vi "onProcessStopped.vi"(8 "error in (no error)":errorcluster, 11 "SystemController":refnum<class "SystemController.lvclass">) -> (0 "error out":errorcluster, 3 "SystemController out":refnum<class "SystemController.lvclass">)   [LabVIEW 2017, in "SystemController.lvclass"]
doc: "JKI State Machine Objects (SMO) 1.3.0.56\nJKI - JKI\nCopyright (c) 2017, JKI"
uses:
  SystemController.lvclass
  Camera/Camera_class/Camera.lvclass
  ImageFacialDetection_class/ImageFacialDetection.lvclass
  <vilib>/JKI/JKI SMO/SMO/SMO.lvclass
panel:
  # "For instructions on how to use the JKI State Machine Objects, examples and video tutorials, visit:\nhttp://jki.net/state-machine-objects/\n\nJKI State Machine Objects™\nhttp://jki.net/state-machine-objects/\nCopyright (C) 2005-2015, JKI <info@jki.net>\nALL RIGHTS RESERVED"
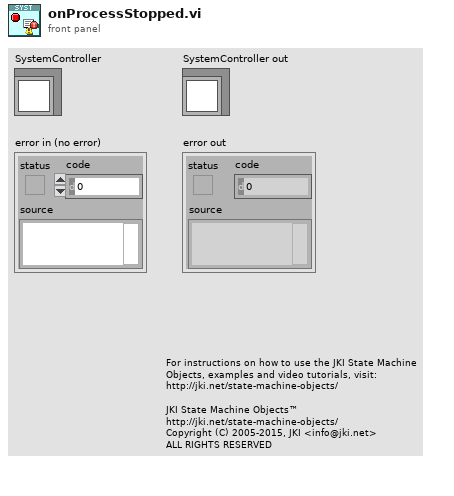
[diagram p1: front panel]
types:
  T1 = typedef "SystemController.lvclass/Dependencies--Cluster.ctl" = cluster{"Camera":refnum<class "Camera.lvclass">, "ImageFacialDetection":refnum<class "ImageFacialDetection.lvclass">}
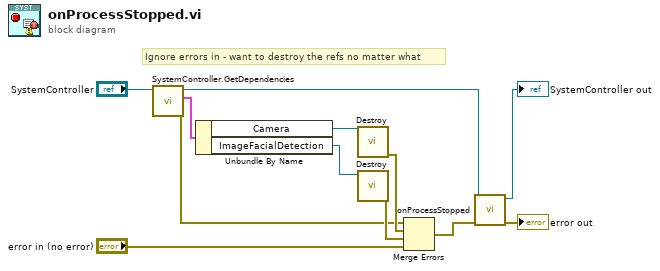
[diagram p0: block diagram]
diagram:
  # "Ignore errors in - want to destroy the refs no matter what"
  n1 = call "SystemController.GetDependencies.vi"("SystemController"="SystemController") -> ("error out"=w2:errorcluster, "Dependencies"=w8:T1, "SystemController out"=w9:refnum<class "SystemController.lvclass">)  [unwired: 8 in]
  n2 = Unbundle By Name(w8) -> ("Camera"=w7:refnum<class "Camera.lvclass">, "ImageFacialDetection"=w6:refnum<class "ImageFacialDetection.lvclass">)
  n3 = call-dynamic "Destroy.vi"("reference in"=w7) -> ("error out"=w3:errorcluster)  [unwired: 9 in, 1 out]
  n4 = call-dynamic "Destroy.vi"("reference in"=w6) -> ("error out"=w4:errorcluster)  [unwired: 9 in, 1 out]
  n5 = Merge Errors(w2, w3, w4, "error in (no error)") -> (w5:errorcluster)
  n6 = call-parent "onProcessStopped.vi"("error in (no error)"=w5, "SMO"=w9) -> ("error out"=→"error out":errorcluster, "SMO out"=→"SystemController out":refnum<class "SystemController.lvclass">)  [unwired: 8 in]
